vi "Motor_Initialization.vi"() -> ()   [LabVIEW 2018]
uses:
  <vilib>/Rock Robotics/WPI/ThirdParty/Phoenix-LabVIEW/Motor Controller/Controls/CTRE_Phoenix_MotorControl_ControlMode.ctl
  <vilib>/Rock Robotics/WPI/ThirdParty/Phoenix-LabVIEW/Motor Controller/Controls/CTRE_Phoenix_MotorControl_FeedbackDevice.ctl
  Global_Variables/Drive_Globals.vi
  Global_Variables/Elevator_Globals.vi
  <vilib>/Rock Robotics/WPI/ThirdParty/Phoenix-LabVIEW/Pigeon IMU/CTRE_PigeonIMU_Open_TalonSRX.vi
  Global_Variables/Climb_Globals.vi
  Global_Variables/Intake_Joint_Globals.vi
  Global_Variables/Intake_Ball_Globals.vi
panel:
  in  "D_Right":dbl
  in  "P_Right":dbl=3.0
  in  "D":dbl
  in  "P_Drive":dbl=3.0
  in  "secondsFromNeutralToFull":dbl
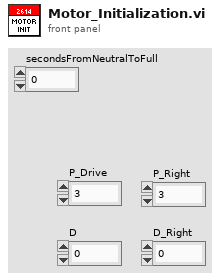
[diagram p1: front panel]
types:
  T1 = typedef "CTRE_Phoenix_MotorControl_FeedbackDevice.ctl" = i8
  T2 = typedef "CTRE_Phoenix_MotorControl_ControlMode.ctl" = u16
  T3 = enum16{"FollowerType_PercentOutput", "FollowerType_AuxOutput1"}
  T4 = typedef "WPI_MotorControlDeviceRef.ctl" = cluster{"DeviceStatus":errorcluster, "Type":T5, "PWM":cluster{"PWM Channel":T6, "DeadBand":T7}, "CAN":cluster{"Device Number":u8, "SetOutput VI Ref":variant, "GetOutput VI Ref":variant, "Enable VI Ref":variant, "Disable VI Ref":variant, "Data":variant}, "Invert":bool, "DIO PWM":cluster{"PWM \"Enable\" Channel":T6, "DIOChannel":T8, "PWM Rate":dbl}}
  T5 = typedef "WPI_MotorControlType.ctl" = enum16{"PWM", "CAN", "DIO PWM"}
  T6 = typedef "FPGA_DIOPWMChannel.ctl" = enum8{"PWM 0", "PWM 1", "PWM 2", "PWM 3", "PWM 4", "PWM 5", "PWM 6", "PWM 7", "PWM 8", "PWM 9", "PWM MXP 0", "PWM MXP 1", "PWM MXP 2", "PWM MXP 3", "PWM MXP 4", "PWM MXP 5", "PWM MXP 6", "PWM MXP 7", "PWM MXP 8", "PWM MXP 9", "Invalid"}
  T7 = typedef "WPI_PWMDeadband.ctl" = cluster{"Name":string, "maxPositivePwm":i32, "minPositivePwm":i32, "centerPwm":i32, "maxNegativePwm":i32, "minNegativePwm":i32, "angularRange":u16}
  T8 = typedef "FPGA_DIOChannel.ctl" = enum8{"DIO 0", "DIO 1", "DIO 2", "DIO 3", "DIO 4", "DIO 5", "DIO 6", "DIO 7", "DIO 8", "DIO 9", "DIO MXP 0", "DIO MXP 1", "DIO MXP 2", "DIO MXP 3", "DIO MXP 4", "DIO MXP 5", "DIO MXP 6", "DIO MXP 7", "DIO MXP 8", "DIO MXP 9", "DIO MXP 10", "DIO MXP 11", "DIO MXP 12", "DIO MXP 13", "DIO MXP 14", "DIO MXP 15", "SPI Port CS1", "SPI Port CS2", "SPI Port CS3", "SPI Port MISO", "SPI Port MOSI", "Invalid"}
  T9 = typedef "CTRE_PigeonIMU_DeviceRef.ctl" = cluster{"DeviceStatus":errorcluster, "Device Number":u8, "Type":T10, "Device ID":u32, "Handle":u64, "UsageFrame":u32, "Library Path":path}
  T10 = typedef "CTRE_PigeonIMU_ConnectionType.ctl" = u32
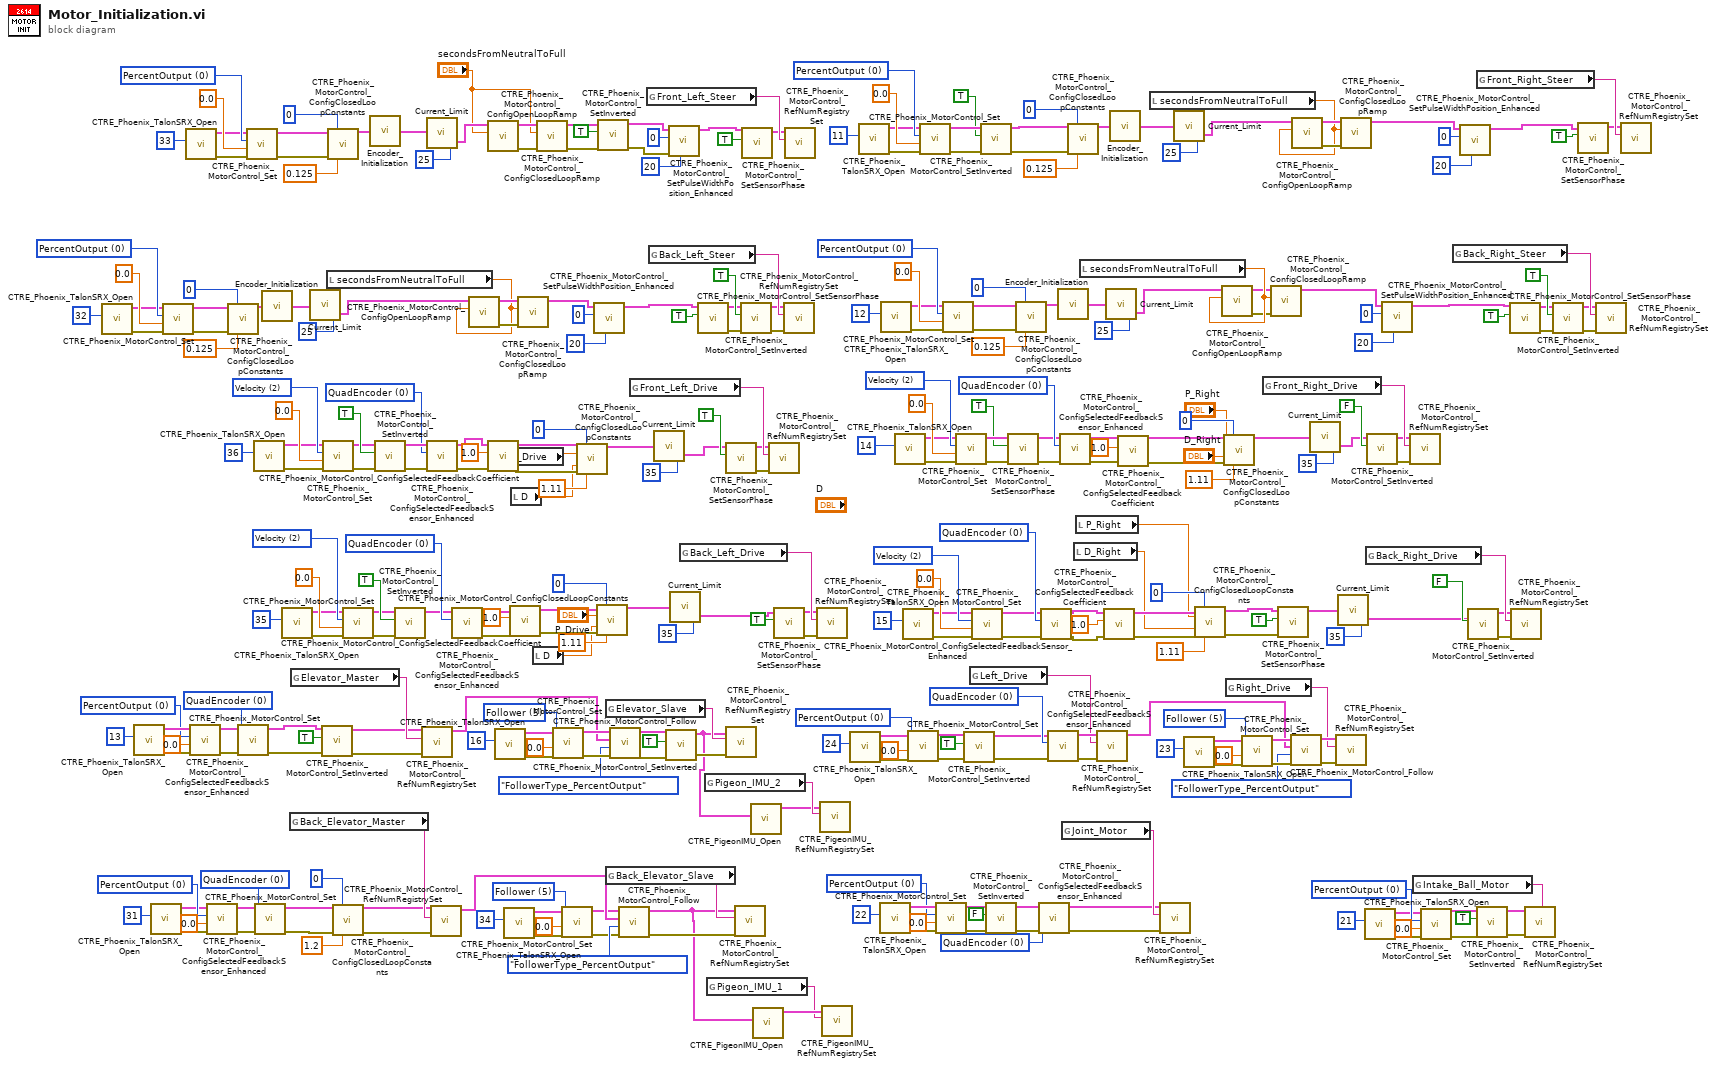
[diagram p0: block diagram]
diagram:
  w60 = T1 0 items=["QuadEncoder"=0, "Analog"=2, "Tachometer"=4, "Pulse Width Encoded Position"=8, "Sensor Sum (S0 + S1)"=9, "Sensor Difference (D0 - D1)"=10, "Remote Source 0"=11, "Remote Source 1"=12, "Software Emulated"=15] ("Feedback Device")
  w109 = T2 0 items=["PercentOutput"=0, "Position"=1, "Velocity"=2, "Current"=3, "Follower"=5, "MotionProfile"=6, "MotionMagic"=7, "MotionProfileArc"=10, "Disabled"=15] ("Control Mode")
  w114 = T2 0 items=["PercentOutput"=0, "Position"=1, "Velocity"=2, "Current"=3, "Follower"=5, "MotionProfile"=6, "MotionMagic"=7, "MotionProfileArc"=10, "Disabled"=15] ("Control Mode")
  w130 = T1 0 items=["QuadEncoder"=0, "Analog"=2, "Tachometer"=4, "Pulse Width Encoded Position"=8, "Sensor Sum (S0 + S1)"=9, "Sensor Difference (D0 - D1)"=10, "Remote Source 0"=11, "Remote Source 1"=12, "Software Emulated"=15] ("Feedback Device")
  w126 = T2 0 items=["PercentOutput"=0, "Position"=1, "Velocity"=2, "Current"=3, "Follower"=5, "MotionProfile"=6, "MotionMagic"=7, "MotionProfileArc"=10, "Disabled"=15] ("Control Mode")
  w125 = T2 5 items=["PercentOutput"=0, "Position"=1, "Velocity"=2, "Current"=3, "Follower"=5, "MotionProfile"=6, "MotionMagic"=7, "MotionProfileArc"=10, "Disabled"=15] ("Control Mode")
  w151 = T1 0 items=["None"=-1, "QuadEncoder"=0, "Analog"=2, "Tachometer"=4, "Pulse Width Encoded Position"=8, "Sensor Sum (S0 + S1)"=9, "Sensor Difference (D0 - D1)"=10, "Remote Source 0"=11, "Remote Source 1"=12, "Software Emulated"=15] ("Feedback Device")
  w154 = T2 0 items=["PercentOutput"=0, "Position"=1, "Velocity"=2, "Current"=3, "Follower"=5, "MotionProfile"=6, "MotionMagic"=7, "MotionProfileArc"=10, "Disabled"=15] ("Control Mode")
  w155 = T2 5 items=["PercentOutput"=0, "Position"=1, "Velocity"=2, "Current"=3, "Follower"=5, "MotionProfile"=6, "MotionMagic"=7, "MotionProfileArc"=10, "Disabled"=15] ("Control Mode")
  w164 = T1 0 items=["QuadEncoder"=0, "Analog"=2, "Tachometer"=4, "Pulse Width Encoded Position"=8, "Sensor Sum (S0 + S1)"=9, "Sensor Difference (D0 - D1)"=10, "Remote Source 0"=11, "Remote Source 1"=12, "Software Emulated"=15] ("Feedback Device")
  w169 = T2 0 items=["PercentOutput"=0, "Position"=1, "Velocity"=2, "Current"=3, "Follower"=5, "MotionProfile"=6, "MotionMagic"=7, "MotionProfileArc"=10, "Disabled"=15] ("Control Mode")
  w170 = T2 5 items=["PercentOutput"=0, "Position"=1, "Velocity"=2, "Current"=3, "Follower"=5, "MotionProfile"=6, "MotionMagic"=7, "MotionProfileArc"=10, "Disabled"=15] ("Control Mode")
  w214 = T1 0 items=["None"=-1, "QuadEncoder"=0, "Analog"=2, "Tachometer"=4, "Pulse Width Encoded Position"=8, "Sensor Sum (S0 + S1)"=9, "Sensor Difference (D0 - D1)"=10, "Remote Source 0"=11, "Remote Source 1"=12, "Software Emulated"=15] ("Feedback Device")
  w222 = T1 0 items=["None"=-1, "QuadEncoder"=0, "Analog"=2, "Tachometer"=4, "Pulse Width Encoded Position"=8, "Sensor Sum (S0 + S1)"=9, "Sensor Difference (D0 - D1)"=10, "Remote Source 0"=11, "Remote Source 1"=12, "Software Emulated"=15] ("Feedback Device")
  w223 = T1 0 items=["None"=-1, "QuadEncoder"=0, "Analog"=2, "Tachometer"=4, "Pulse Width Encoded Position"=8, "Sensor Sum (S0 + S1)"=9, "Sensor Difference (D0 - D1)"=10, "Remote Source 0"=11, "Remote Source 1"=12, "Software Emulated"=15] ("Feedback Device")
  w225 = T1 0 items=["None"=-1, "QuadEncoder"=0, "Analog"=2, "Tachometer"=4, "Pulse Width Encoded Position"=8, "Sensor Sum (S0 + S1)"=9, "Sensor Difference (D0 - D1)"=10, "Remote Source 0"=11, "Remote Source 1"=12, "Software Emulated"=15] ("Feedback Device")
  w246 = T2 2 items=["PercentOutput"=0, "Position"=1, "Velocity"=2, "Current"=3, "Follower"=5, "MotionProfile"=6, "MotionMagic"=7, "MotionMagicArc"=8, "MotionProfileArc"=10, "Disabled"=15] ("Control Mode")
  w251 = T2 2 items=["PercentOutput"=0, "Position"=1, "Velocity"=2, "Current"=3, "Follower"=5, "MotionProfile"=6, "MotionMagic"=7, "MotionMagicArc"=8, "MotionProfileArc"=10, "Disabled"=15] ("Control Mode")
  w256 = T2 2 items=["PercentOutput"=0, "Position"=1, "Velocity"=2, "Current"=3, "Follower"=5, "MotionProfile"=6, "MotionMagic"=7, "MotionMagicArc"=8, "MotionProfileArc"=10, "Disabled"=15] ("Control Mode")
  w261 = T2 2 items=["PercentOutput"=0, "Position"=1, "Velocity"=2, "Current"=3, "Follower"=5, "MotionProfile"=6, "MotionMagic"=7, "MotionMagicArc"=8, "MotionProfileArc"=10, "Disabled"=15] ("Control Mode")
  w293 = T2 0 items=["PercentOutput"=0, "Position"=1, "Velocity"=2, "Current"=3, "Follower"=5, "MotionProfile"=6, "MotionMagic"=7, "MotionMagicArc"=8, "MotionProfileArc"=10, "Disabled"=15] ("Control Mode")
  w302 = T2 0 items=["PercentOutput"=0, "Position"=1, "Velocity"=2, "Current"=3, "Follower"=5, "MotionProfile"=6, "MotionMagic"=7, "MotionMagicArc"=8, "MotionProfileArc"=10, "Disabled"=15] ("Control Mode")
  w311 = T2 0 items=["PercentOutput"=0, "Position"=1, "Velocity"=2, "Current"=3, "Follower"=5, "MotionProfile"=6, "MotionMagic"=7, "MotionMagicArc"=8, "MotionProfileArc"=10, "Disabled"=15] ("Control Mode")
  w320 = T2 0 items=["PercentOutput"=0, "Position"=1, "Velocity"=2, "Current"=3, "Follower"=5, "MotionProfile"=6, "MotionMagic"=7, "MotionMagicArc"=8, "MotionProfileArc"=10, "Disabled"=15] ("Control Mode")
  n1 = call <vilib>:"CTRE_Phoenix_TalonSRX_Open.vi"("Device Number"=u8 32) -> ("error out"=w313:errorcluster, "CAN Talon SRX Ref"=w310:T4)  [unwired: 9 in]
  n2 = call <vilib>:"CTRE_Phoenix_TalonSRX_Open.vi"("Device Number"=u8 13) -> ("error out"=w176:errorcluster, "CAN Talon SRX Ref"=w175:T4)  [unwired: 9 in]
  n3 = call <vilib>:"CTRE_Phoenix_TalonSRX_Open.vi"("Device Number"=u8 31) -> ("error out"=w119:errorcluster, "CAN Talon SRX Ref"=w120:T4)  [unwired: 9 in]
  n4 = call <vilib>:"CTRE_Phoenix_MotorControl_Set.vi"("error in (no error)"=w313, "Output"=0.0, "Control Mode"=w311, "PhoenixMotorControlDevRef"=w310) -> ("error out"=w315:errorcluster, "PhoenixMotorControlDevRef"=w314:T4)  [unwired: 6 in]
  n5 = call <vilib>:"CTRE_Phoenix_TalonSRX_Open.vi"("Device Number"=u8 33) -> ("error out"=w322:errorcluster, "CAN Talon SRX Ref"=w319:T4)  [unwired: 9 in]
  n6 = call <vilib>:"CTRE_Phoenix_MotorControl_Set.vi"("error in (no error)"=w176, "Output"=0.0, "Control Mode"=w169, "PhoenixMotorControlDevRef"=w175) -> ("error out"=w166:errorcluster, "PhoenixMotorControlDevRef"=w165:T4)  [unwired: 6 in]
  n7 = call <vilib>:"CTRE_Phoenix_MotorControl_Set.vi"("error in (no error)"=w119, "Output"=0.0, "Control Mode"=w126, "PhoenixMotorControlDevRef"=w120) -> ("error out"=w128:errorcluster, "PhoenixMotorControlDevRef"=w129:T4)  [unwired: 6 in]
  n8 = call <vilib>:"CTRE_Phoenix_MotorControl_ConfigClosedLoopConstants.vi"("PhoenixMotorControlDevRef"=w314, "slotIdx"=0, "error in (no error)"=w315, "F"=0.125) -> ("PhoenixMotorControlDevRef"=w279:T4)  [unwired: 10 in, 1 out]
  n9 = call <vilib>:"CTRE_Phoenix_MotorControl_ConfigSelectedFeedbackSensor_Enhanced.vi"("error in (no error)"=w166, "Feedback Device"=w164, "PhoenixMotorControlDevRef"=w165) -> ("error out"=w94:errorcluster, "PhoenixMotorControlDevRef"=w95:T4)  [unwired: 7 in]
  n10 = call <vilib>:"CTRE_Phoenix_MotorControl_Set.vi"("error in (no error)"=w322, "Output"=0.0, "Control Mode"=w320, "PhoenixMotorControlDevRef"=w319) -> ("error out"=w324:errorcluster, "PhoenixMotorControlDevRef"=w323:T4)  [unwired: 6 in]
  n11 = call <vilib>:"CTRE_Phoenix_TalonSRX_Open.vi"("Device Number"=u8 36) -> ("error out"=w206:errorcluster, "CAN Talon SRX Ref"=w207:T4)  [unwired: 9 in]
  n12 = call <vilib>:"CTRE_Phoenix_MotorControl_ConfigSelectedFeedbackSensor_Enhanced.vi"("error in (no error)"=w128, "Feedback Device"=w130, "PhoenixMotorControlDevRef"=w129) -> ("error out"=w86:errorcluster, "PhoenixMotorControlDevRef"=w87:T4)  [unwired: 7 in]
  n13 = call "Encoder_Initialization.vi"("Ref In"=w279) -> ("Ref Out"=w78:T4)  [unwired: 1 in]
  n14 = call <vilib>:"CTRE_Phoenix_TalonSRX_Open.vi"("Device Number"=u8 35) -> ("error out"=w248:errorcluster, "CAN Talon SRX Ref"=w245:T4)  [unwired: 9 in]
  n15 = global read "Climb_Globals.vi" "Back_Elevator_Master"() -> (w118:string)
  n16 = global read "Elevator_Globals.vi" "Elevator_Master"() -> (w167:string)
  n17 = call "Current_Limit.vi"("Ref In"=w78, "Current_Limit"=25) -> ("Ref Out"=w38:T4)
  n18 = call <vilib>:"CTRE_Phoenix_MotorControl_SetInverted.vi"("error in (no error)"=w94, "Invert?"=TRUE, "PhoenixMotorControlDevRef"=w95) -> ("error out"=w92:errorcluster, "PhoenixMotorControlDevRef"=w93:T4)  [unwired: 7 in]
  n19 = call <vilib>:"CTRE_Phoenix_MotorControl_Set.vi"("error in (no error)"=w206, "Output"=0.0, "Control Mode"=w251, "PhoenixMotorControlDevRef"=w207) -> ("error out"=w241:errorcluster, "PhoenixMotorControlDevRef"=w242:T4)  [unwired: 6 in]
  n20 = local read "secondsFromNeutralToFull"() -> (w39:dbl)
  n21 = call <vilib>:"CTRE_Phoenix_MotorControl_ConfigClosedLoopConstants.vi"("PhoenixMotorControlDevRef"=w323, "slotIdx"=0, "error in (no error)"=w324, "F"=0.125) -> ("PhoenixMotorControlDevRef"=w282:T4)  [unwired: 10 in, 1 out]
  n22 = call <vilib>:"CTRE_Phoenix_MotorControl_ConfigClosedLoopConstants.vi"("PhoenixMotorControlDevRef"=w87, "slotIdx"=0, "error in (no error)"=w86, "F"=1.2) -> ("PhoenixMotorControlDevRef"=w85:T4, "error out"=w84:errorcluster)  [unwired: 10 in]
  n23 = call <vilib>:"CTRE_Phoenix_MotorControl_Set.vi"("error in (no error)"=w248, "Output"=0.0, "Control Mode"=w246, "PhoenixMotorControlDevRef"=w245) -> ("error out"=w238:errorcluster, "PhoenixMotorControlDevRef"=w239:T4)  [unwired: 6 in]
  n24 = call "Encoder_Initialization.vi"("Ref In"=w282) -> ("Ref Out"=w77:T4)  [unwired: 1 in]
  n25 = call <vilib>:"CTRE_Phoenix_MotorControl_SetInverted.vi"("error in (no error)"=w241, "Invert?"=TRUE, "PhoenixMotorControlDevRef"=w242) -> ("error out"=w218:errorcluster, "PhoenixMotorControlDevRef"=w217:T4)  [unwired: 7 in]
  n26 = call <vilib>:"CTRE_Phoenix_MotorControl_SetInverted.vi"("error in (no error)"=w238, "Invert?"=TRUE, "PhoenixMotorControlDevRef"=w239) -> ("PhoenixMotorControlDevRef"=w224:T4)  [unwired: 7 in, 1 out]
  n27 = call <vilib>:"CTRE_Phoenix_MotorControl_RefNumRegistrySet.vi"("error in (no error)"=w92, "refnum name"=w167, "PhoenixMotorControlDevRef"=w93) -> ("PhoenixMotorControlDevRef"=w139:T4)  [unwired: 7 in, 1 out]
  n28 = call "Current_Limit.vi"("Ref In"=w77, "Current_Limit"=25) -> ("Ref Out"=w43:T4)
  n29 = call <vilib>:"CTRE_Phoenix_MotorControl_ConfigSelectedFeedbackSensor_Enhanced.vi"("error in (no error)"=w218, "Feedback Device"=w214, "PhoenixMotorControlDevRef"=w217) -> ("error out"=w181:errorcluster, "PhoenixMotorControlDevRef"=w182:T4)  [unwired: 7 in]
  n30 = call <vilib>:"CTRE_Phoenix_MotorControl_RefNumRegistrySet.vi"("error in (no error)"=w84, "refnum name"=w118, "PhoenixMotorControlDevRef"=w85) -> ("PhoenixMotorControlDevRef"=w136:T4)  [unwired: 7 in, 1 out]
  n31 = call <vilib>:"CTRE_Phoenix_MotorControl_ConfigSelectedFeedbackSensor_Enhanced.vi"("Feedback Device"=w225, "PhoenixMotorControlDevRef"=w224) -> ("error out"=w208:errorcluster, "PhoenixMotorControlDevRef"=w209:T4)  [unwired: 8 in]
  n32 = call <vilib>:"CTRE_Phoenix_MotorControl_ConfigOpenLoopRamp.vi"("secondsFromNeutralToFull"=w39, "PhoenixMotorControlDevRef"=w38) -> ("error out"=w41:errorcluster, "PhoenixMotorControlDevRef"=w40:T4)  [unwired: 8 in]
  n33 = call <vilib>:"CTRE_Phoenix_MotorControl_ConfigOpenLoopRamp.vi"("secondsFromNeutralToFull"="secondsFromNeutralToFull", "PhoenixMotorControlDevRef"=w43) -> ("error out"=w44:errorcluster, "PhoenixMotorControlDevRef"=w45:T4)  [unwired: 8 in]
  n34 = call <vilib>:"CTRE_Phoenix_MotorControl_ConfigSelectedFeedbackCoefficient.vi"("error in (no error)"=w181, "coefficient"=1.0, "PhoenixMotorControlDevRef"=w182) -> ("error out"=w177:errorcluster, "PhoenixMotorControlDevRef"=w178:T4)  [unwired: 7 in]
  n35 = call <vilib>:"CTRE_Phoenix_TalonSRX_Open.vi"("Device Number"=u8 16) -> ("error out"=w174:errorcluster, "CAN Talon SRX Ref"=w173:T4)  [unwired: 9 in]
  n36 = local read "P_Drive"() -> (w12:dbl)
  n37 = call <vilib>:"CTRE_Phoenix_TalonSRX_Open.vi"("Device Number"=u8 34) -> ("error out"=w121:errorcluster, "CAN Talon SRX Ref"=w122:T4)  [unwired: 9 in]
  n38 = call <vilib>:"CTRE_Phoenix_MotorControl_ConfigSelectedFeedbackCoefficient.vi"("error in (no error)"=w208, "coefficient"=1.0, "PhoenixMotorControlDevRef"=w209) -> ("error out"=w184:errorcluster, "PhoenixMotorControlDevRef"=w185:T4)  [unwired: 7 in]
  n39 = local read "D"() -> (w5:dbl)
  n40 = call <vilib>:"CTRE_Phoenix_MotorControl_ConfigClosedLoopRamp.vi"("error in (no error)"=w41, "secondsFromNeutralToFull"=w39, "PhoenixMotorControlDevRef"=w40) -> ("PhoenixMotorControlDevRef"=w37:T4)  [unwired: 7 in, 1 out]
  n41 = local read "D"() -> (w6:dbl)
  n42 = call <vilib>:"CTRE_Phoenix_MotorControl_ConfigClosedLoopRamp.vi"("error in (no error)"=w44, "secondsFromNeutralToFull"="secondsFromNeutralToFull", "PhoenixMotorControlDevRef"=w45) -> ("error out"=w25:errorcluster, "PhoenixMotorControlDevRef"=w26:T4)  [unwired: 7 in]
  n43 = call <vilib>:"CTRE_Phoenix_MotorControl_Set.vi"("error in (no error)"=w174, "Output"=0.0, "Control Mode"=w170, "PhoenixMotorControlDevRef"=w173) -> ("error out"=w172:errorcluster, "PhoenixMotorControlDevRef"=w171:T4)  [unwired: 6 in]
  n44 = call <vilib>:"CTRE_Phoenix_MotorControl_Set.vi"("error in (no error)"=w121, "Output"=0.0, "Control Mode"=w125, "PhoenixMotorControlDevRef"=w122) -> ("error out"=w123:errorcluster, "PhoenixMotorControlDevRef"=w124:T4)  [unwired: 6 in]
  n45 = call <vilib>:"CTRE_Phoenix_MotorControl_ConfigClosedLoopConstants.vi"("PhoenixMotorControlDevRef"=w178, "slotIdx"=0, "P"=w12, "D"=w5, "error in (no error)"=w177, "F"=1.11) -> ("PhoenixMotorControlDevRef"=w70:T4)  [unwired: 8 in, 1 out]
  n46 = call <vilib>:"CTRE_Phoenix_MotorControl_SetPulseWidthPosition_Enhanced.vi"("timeoutMs"=u32 20, "New Position"=0, "PhoenixMotorControlDevRef"=w37) -> ("PhoenixMotorControlDevRef"=w66:T4)  [unwired: 7 in, 1 out]
  n47 = call <vilib>:"CTRE_Phoenix_MotorControl_ConfigClosedLoopConstants.vi"("PhoenixMotorControlDevRef"=w185, "slotIdx"=0, "P"="P_Drive", "D"=w6, "error in (no error)"=w184, "F"=1.11) -> ("PhoenixMotorControlDevRef"=w72:T4)  [unwired: 8 in, 1 out]
  n48 = call <vilib>:"CTRE_Phoenix_MotorControl_SetInverted.vi"("error in (no error)"=w25, "Invert?"=TRUE, "PhoenixMotorControlDevRef"=w26) -> ("error out"=w23:errorcluster, "PhoenixMotorControlDevRef"=w24:T4)  [unwired: 7 in]
  n49 = global read "Elevator_Globals.vi" "Elevator_Slave"() -> (w168:string)
  n50 = global read "Climb_Globals.vi" "Back_Elevator_Slave"() -> (w117:string)
  n51 = call <vilib>:"CTRE_Phoenix_MotorControl_Follow.vi"("error in (no error)"=w172, "FollowerType"=T3."FollowerType_PercentOutput", "Master Controller to Follow"=w139, "PhoenixMotorControlDevRef"=w171) -> ("error out"=w88:errorcluster, "PhoenixMotorControlDevRef"=w90:T4)  [unwired: 6 in]
  n52 = call <vilib>:"CTRE_Phoenix_MotorControl_Follow.vi"("error in (no error)"=w123, "FollowerType"=T3."FollowerType_PercentOutput", "Master Controller to Follow"=w136, "PhoenixMotorControlDevRef"=w124) -> ("error out"=w127:errorcluster, "PhoenixMotorControlDevRef"=w46:T4)  [unwired: 6 in]
  n53 = global read "Drive_Globals.vi" "Front_Left_Drive"() -> (w253:string)
  n54 = global read "Drive_Globals.vi" "Front_Left_Steer"() -> (w286:string)
  n55 = global read "Drive_Globals.vi" "Back_Left_Steer"() -> (w317:string)
  n56 = call "Current_Limit.vi"("Ref In"=w70, "Current_Limit"=35) -> ("Ref Out"=w69:T4)
  n57 = call <vilib>:"CTRE_Phoenix_MotorControl_SetInverted.vi"("error in (no error)"=w88, "Invert?"=TRUE, "PhoenixMotorControlDevRef"=w90) -> ("error out"=w89:errorcluster, "PhoenixMotorControlDevRef"=w49:T4)  [unwired: 7 in]
  n58 = call <vilib>:"CTRE_Phoenix_MotorControl_SetPulseWidthPosition_Enhanced.vi"("timeoutMs"=u32 20, "error in (no error)"=w23, "New Position"=0, "PhoenixMotorControlDevRef"=w24) -> ("PhoenixMotorControlDevRef"=w65:T4)  [unwired: 6 in, 1 out]
  n59 = call "Current_Limit.vi"("Ref In"=w72, "Current_Limit"=35) -> ("Ref Out"=w71:T4)
  n60 = global read "Drive_Globals.vi" "Back_Left_Drive"() -> (w249:string)
  n61 = call <vilib>:"CTRE_Phoenix_MotorControl_SetSensorPhase.vi"("PhaseSensor"=TRUE, "PhoenixMotorControlDevRef"=w66) -> ("error out"=w266:errorcluster, "PhoenixMotorControlDevRef"=w267:T4)  [unwired: 8 in]
  n62 = global read "Drive_Globals.vi" "Pigeon_IMU_2"() -> (w51:string)
  n63 = global read "Drive_Globals.vi" "Pigeon_IMU_1"() -> (w47:string)
  n64 = call <vilib>:"CTRE_Phoenix_MotorControl_SetSensorPhase.vi"("PhaseSensor"=TRUE, "PhoenixMotorControlDevRef"=w69) -> ("error out"=w215:errorcluster, "PhoenixMotorControlDevRef"=w216:T4)  [unwired: 8 in]
  n65 = call <vilib>:"CTRE_Phoenix_MotorControl_RefNumRegistrySet.vi"("error in (no error)"=w89, "refnum name"=w168, "PhoenixMotorControlDevRef"=w49) -> ()  [unwired: 7 in, 2 out]
  n66 = call <vilib>:"CTRE_Phoenix_MotorControl_RefNumRegistrySet.vi"("error in (no error)"=w127, "refnum name"=w117, "PhoenixMotorControlDevRef"=w46) -> ()  [unwired: 7 in, 2 out]
  n67 = call <vilib>:"CTRE_Phoenix_MotorControl_SetInverted.vi"("error in (no error)"=w266, "Invert?"=TRUE, "PhoenixMotorControlDevRef"=w267) -> ("error out"=w265:errorcluster, "PhoenixMotorControlDevRef"=w264:T4)  [unwired: 7 in]
  n68 = call <vilib>:"CTRE_Phoenix_MotorControl_SetSensorPhase.vi"("PhaseSensor"=TRUE, "PhoenixMotorControlDevRef"=w65) -> ("PhoenixMotorControlDevRef"=w277:T4)  [unwired: 8 in, 1 out]
  n69 = call-poly <vilib>:"CTRE_PigeonIMU_Open.vi"("CAN Talon SRX Ref"=w49) -> ("PigeonIMUDevRef"=w50:T9)  [unwired: 9 in, 1 out]
  n70 = call-poly <vilib>:"CTRE_PigeonIMU_Open.vi"("CAN Talon SRX Ref"=w46) -> ("PigeonIMUDevRef"=w48:T9)  [unwired: 9 in, 1 out]
  n71 = call <vilib>:"CTRE_Phoenix_MotorControl_RefNumRegistrySet.vi"("error in (no error)"=w215, "refnum name"=w253, "PhoenixMotorControlDevRef"=w216) -> ()  [unwired: 7 in, 2 out]
  n72 = call <vilib>:"CTRE_Phoenix_MotorControl_SetSensorPhase.vi"("PhaseSensor"=TRUE, "PhoenixMotorControlDevRef"=w71) -> ("error out"=w230:errorcluster, "PhoenixMotorControlDevRef"=w231:T4)  [unwired: 8 in]
  n73 = call <vilib>:"CTRE_Phoenix_MotorControl_RefNumRegistrySet.vi"("error in (no error)"=w265, "refnum name"=w317, "PhoenixMotorControlDevRef"=w264) -> ()  [unwired: 7 in, 2 out]
  n74 = call <vilib>:"CTRE_Phoenix_MotorControl_RefNumRegistrySet.vi"("refnum name"=w286, "PhoenixMotorControlDevRef"=w277) -> ()  [unwired: 8 in, 2 out]
  n75 = call <vilib>:"CTRE_Phoenix_MotorControl_RefNumRegistrySet.vi"("error in (no error)"=w230, "refnum name"=w249, "PhoenixMotorControlDevRef"=w231) -> ()  [unwired: 7 in, 2 out]
  n76 = call <vilib>:"CTRE_PigeonIMU_RefNumRegistrySet.vi"("refnum name"=w51, "PigeonIMUDevRef"=w50) -> ()  [unwired: 8 in, 2 out]
  n77 = call <vilib>:"CTRE_PigeonIMU_RefNumRegistrySet.vi"("refnum name"=w47, "PigeonIMUDevRef"=w48) -> ()  [unwired: 8 in, 2 out]
  n78 = call <vilib>:"CTRE_Phoenix_TalonSRX_Open.vi"("Device Number"=u8 24) -> ("error out"=w159:errorcluster, "CAN Talon SRX Ref"=w160:T4)  [unwired: 9 in]
  n79 = call <vilib>:"CTRE_Phoenix_TalonSRX_Open.vi"("Device Number"=u8 11) -> ("error out"=w304:errorcluster, "CAN Talon SRX Ref"=w301:T4)  [unwired: 9 in]
  n80 = call <vilib>:"CTRE_Phoenix_TalonSRX_Open.vi"("Device Number"=u8 22) -> ("error out"=w116:errorcluster, "CAN Talon SRX Ref"=w115:T4)  [unwired: 9 in]
  n81 = call <vilib>:"CTRE_Phoenix_TalonSRX_Open.vi"("Device Number"=u8 12) -> ("error out"=w295:errorcluster, "CAN Talon SRX Ref"=w292:T4)  [unwired: 9 in]
  n82 = call <vilib>:"CTRE_Phoenix_TalonSRX_Open.vi"("Device Number"=u8 14) -> ("error out"=w211:errorcluster, "CAN Talon SRX Ref"=w212:T4)  [unwired: 9 in]
  n83 = call <vilib>:"CTRE_Phoenix_TalonSRX_Open.vi"("Device Number"=u8 15) -> ("error out"=w258:errorcluster, "CAN Talon SRX Ref"=w255:T4)  [unwired: 9 in]
  n84 = call <vilib>:"CTRE_Phoenix_MotorControl_Set.vi"("error in (no error)"=w159, "Output"=0.0, "Control Mode"=w154, "PhoenixMotorControlDevRef"=w160) -> ("error out"=w101:errorcluster, "PhoenixMotorControlDevRef"=w100:T4)  [unwired: 6 in]
  n85 = call <vilib>:"CTRE_Phoenix_MotorControl_Set.vi"("error in (no error)"=w304, "Output"=0.0, "Control Mode"=w302, "PhoenixMotorControlDevRef"=w301) -> ("error out"=w306:errorcluster, "PhoenixMotorControlDevRef"=w305:T4)  [unwired: 6 in]
  n86 = call <vilib>:"CTRE_Phoenix_MotorControl_Set.vi"("error in (no error)"=w116, "Output"=0.0, "Control Mode"=w114, "PhoenixMotorControlDevRef"=w115) -> ("error out"=w104:errorcluster, "PhoenixMotorControlDevRef"=w103:T4)  [unwired: 6 in]
  n87 = call <vilib>:"CTRE_Phoenix_MotorControl_Set.vi"("error in (no error)"=w295, "Output"=0.0, "Control Mode"=w293, "PhoenixMotorControlDevRef"=w292) -> ("error out"=w297:errorcluster, "PhoenixMotorControlDevRef"=w296:T4)  [unwired: 6 in]
  n88 = call <vilib>:"CTRE_Phoenix_MotorControl_Set.vi"("error in (no error)"=w211, "Output"=0.0, "Control Mode"=w261, "PhoenixMotorControlDevRef"=w212) -> ("error out"=w228:errorcluster, "PhoenixMotorControlDevRef"=w227:T4)  [unwired: 6 in]
  n89 = call <vilib>:"CTRE_Phoenix_MotorControl_SetInverted.vi"("error in (no error)"=w101, "Invert?"=TRUE, "PhoenixMotorControlDevRef"=w100) -> ("error out"=w98:errorcluster, "PhoenixMotorControlDevRef"=w99:T4)  [unwired: 7 in]
  n90 = global read "Climb_Globals.vi" "Left_Drive"() -> (w142:string)
  n91 = call <vilib>:"CTRE_Phoenix_MotorControl_Set.vi"("error in (no error)"=w258, "Output"=0.0, "Control Mode"=w256, "PhoenixMotorControlDevRef"=w255) -> ("error out"=w196:errorcluster, "PhoenixMotorControlDevRef"=w197:T4)  [unwired: 6 in]
  n92 = call <vilib>:"CTRE_Phoenix_MotorControl_SetInverted.vi"("error in (no error)"=w306, "Invert?"=TRUE, "PhoenixMotorControlDevRef"=w305) -> ("error out"=w284:errorcluster, "PhoenixMotorControlDevRef"=w283:T4)  [unwired: 7 in]
  n93 = call <vilib>:"CTRE_Phoenix_MotorControl_SetInverted.vi"("error in (no error)"=w104, "Invert?"=FALSE, "PhoenixMotorControlDevRef"=w103) -> ("error out"=w64:errorcluster, "PhoenixMotorControlDevRef"=w63:T4)  [unwired: 7 in]
  n94 = call <vilib>:"CTRE_Phoenix_MotorControl_SetSensorPhase.vi"("error in (no error)"=w228, "PhaseSensor"=TRUE, "PhoenixMotorControlDevRef"=w227) -> ("error out"=w220:errorcluster, "PhoenixMotorControlDevRef"=w221:T4)  [unwired: 7 in]
  n95 = call <vilib>:"CTRE_Phoenix_MotorControl_ConfigClosedLoopConstants.vi"("PhoenixMotorControlDevRef"=w296, "slotIdx"=0, "error in (no error)"=w297, "F"=0.125) -> ("PhoenixMotorControlDevRef"=w281:T4)  [unwired: 10 in, 1 out]
  n96 = call <vilib>:"CTRE_Phoenix_MotorControl_ConfigSelectedFeedbackSensor_Enhanced.vi"("error in (no error)"=w64, "Feedback Device"=w60, "PhoenixMotorControlDevRef"=w63) -> ("error out"=w61:errorcluster, "PhoenixMotorControlDevRef"=w62:T4)  [unwired: 7 in]
  n97 = call <vilib>:"CTRE_Phoenix_MotorControl_ConfigSelectedFeedbackSensor_Enhanced.vi"("error in (no error)"=w196, "Feedback Device"=w223, "PhoenixMotorControlDevRef"=w197) -> ("error out"=w194:errorcluster, "PhoenixMotorControlDevRef"=w195:T4)  [unwired: 7 in]
  n98 = call <vilib>:"CTRE_Phoenix_MotorControl_ConfigSelectedFeedbackSensor_Enhanced.vi"("error in (no error)"=w98, "Feedback Device"=w151, "PhoenixMotorControlDevRef"=w99) -> ("error out"=w146:errorcluster, "PhoenixMotorControlDevRef"=w145:T4)  [unwired: 7 in]
  n99 = call "Encoder_Initialization.vi"("Ref In"=w281) -> ("Ref Out"=w80:T4)  [unwired: 1 in]
  n100 = call <vilib>:"CTRE_Phoenix_MotorControl_ConfigSelectedFeedbackSensor_Enhanced.vi"("error in (no error)"=w220, "Feedback Device"=w222, "PhoenixMotorControlDevRef"=w221) -> ("error out"=w203:errorcluster, "PhoenixMotorControlDevRef"=w204:T4)  [unwired: 7 in]
  n101 = global read "Intake_Joint_Globals.vi" "Joint_Motor"() -> (w106:string)
  n102 = call <vilib>:"CTRE_Phoenix_MotorControl_ConfigClosedLoopConstants.vi"("PhoenixMotorControlDevRef"=w283, "slotIdx"=0, "error in (no error)"=w284, "F"=0.125) -> ("PhoenixMotorControlDevRef"=w280:T4)  [unwired: 10 in, 1 out]
  n103 = local read "D_Right"() -> (w2:dbl)
  n104 = local read "P_Right"() -> (w1:dbl)
  n105 = local read "secondsFromNeutralToFull"() -> (w36:dbl)
  n106 = call <vilib>:"CTRE_Phoenix_MotorControl_RefNumRegistrySet.vi"("error in (no error)"=w146, "refnum name"=w142, "PhoenixMotorControlDevRef"=w145) -> ("PhoenixMotorControlDevRef"=w140:T4)  [unwired: 7 in, 1 out]
  n107 = call <vilib>:"CTRE_Phoenix_MotorControl_ConfigSelectedFeedbackCoefficient.vi"("error in (no error)"=w194, "coefficient"=1.0, "PhoenixMotorControlDevRef"=w195) -> ("error out"=w190:errorcluster, "PhoenixMotorControlDevRef"=w191:T4)  [unwired: 7 in]
  n108 = call "Current_Limit.vi"("Ref In"=w80, "Current_Limit"=25) -> ("Ref Out"=w33:T4)
  n109 = call "Encoder_Initialization.vi"("Ref In"=w280) -> ("Ref Out"=w79:T4)  [unwired: 1 in]
  n110 = call <vilib>:"CTRE_Phoenix_MotorControl_ConfigSelectedFeedbackCoefficient.vi"("error in (no error)"=w203, "coefficient"=1.0, "PhoenixMotorControlDevRef"=w204) -> ("error out"=w199:errorcluster, "PhoenixMotorControlDevRef"=w200:T4)  [unwired: 7 in]
  n111 = local read "secondsFromNeutralToFull"() -> (w29:dbl)
  n112 = call <vilib>:"CTRE_Phoenix_MotorControl_RefNumRegistrySet.vi"("error in (no error)"=w61, "refnum name"=w106, "PhoenixMotorControlDevRef"=w62) -> ()  [unwired: 7 in, 2 out]
  n113 = call "Current_Limit.vi"("Ref In"=w79, "Current_Limit"=25) -> ("Ref Out"=w28:T4)
  n114 = call <vilib>:"CTRE_Phoenix_TalonSRX_Open.vi"("Device Number"=u8 23) -> ("error out"=w158:errorcluster, "CAN Talon SRX Ref"=w157:T4)  [unwired: 9 in]
  n115 = call <vilib>:"CTRE_Phoenix_MotorControl_ConfigClosedLoopConstants.vi"("PhoenixMotorControlDevRef"=w191, "slotIdx"=0, "P"=w1, "D"=w2, "error in (no error)"=w190, "F"=1.11) -> ("PhoenixMotorControlDevRef"=w188:T4, "error out"=w189:errorcluster)  [unwired: 8 in]
  n116 = call <vilib>:"CTRE_Phoenix_MotorControl_ConfigOpenLoopRamp.vi"("secondsFromNeutralToFull"=w36, "PhoenixMotorControlDevRef"=w33) -> ("error out"=w34:errorcluster, "PhoenixMotorControlDevRef"=w35:T4)  [unwired: 8 in]
  n117 = call <vilib>:"CTRE_Phoenix_MotorControl_ConfigClosedLoopConstants.vi"("PhoenixMotorControlDevRef"=w200, "slotIdx"=0, "P"="P_Right", "D"="D_Right", "error in (no error)"=w199, "F"=1.11) -> ("PhoenixMotorControlDevRef"=w74:T4)  [unwired: 8 in, 1 out]
  n118 = global read "Climb_Globals.vi" "Right_Drive"() -> (w141:string)
  n119 = call <vilib>:"CTRE_Phoenix_MotorControl_Set.vi"("error in (no error)"=w158, "Output"=0.0, "Control Mode"=w155, "PhoenixMotorControlDevRef"=w157) -> ("error out"=w150:errorcluster, "PhoenixMotorControlDevRef"=w149:T4)  [unwired: 6 in]
  n120 = global read "Drive_Globals.vi" "Front_Right_Drive"() -> (w263:string)
  n121 = call <vilib>:"CTRE_Phoenix_MotorControl_ConfigClosedLoopRamp.vi"("error in (no error)"=w34, "secondsFromNeutralToFull"=w36, "PhoenixMotorControlDevRef"=w35) -> ("PhoenixMotorControlDevRef"=w32:T4)  [unwired: 7 in, 1 out]
  n122 = call <vilib>:"CTRE_Phoenix_MotorControl_SetSensorPhase.vi"("error in (no error)"=w189, "PhaseSensor"=TRUE, "PhoenixMotorControlDevRef"=w188) -> ("PhoenixMotorControlDevRef"=w76:T4)  [unwired: 7 in, 1 out]
  n123 = call <vilib>:"CTRE_Phoenix_MotorControl_Follow.vi"("error in (no error)"=w150, "FollowerType"=T3."FollowerType_PercentOutput", "Master Controller to Follow"=w140, "PhoenixMotorControlDevRef"=w149) -> ("error out"=w144:errorcluster, "PhoenixMotorControlDevRef"=w143:T4)  [unwired: 6 in]
  n124 = call <vilib>:"CTRE_Phoenix_MotorControl_ConfigOpenLoopRamp.vi"("secondsFromNeutralToFull"=w29, "PhoenixMotorControlDevRef"=w28) -> ("error out"=w31:errorcluster, "PhoenixMotorControlDevRef"=w30:T4)  [unwired: 8 in]
  n125 = call "Current_Limit.vi"("Ref In"=w74, "Current_Limit"=35) -> ("Ref Out"=w73:T4)
  n126 = call <vilib>:"CTRE_Phoenix_MotorControl_RefNumRegistrySet.vi"("error in (no error)"=w144, "refnum name"=w141, "PhoenixMotorControlDevRef"=w143) -> ()  [unwired: 7 in, 2 out]
  n127 = call "Current_Limit.vi"("Ref In"=w76, "Current_Limit"=35) -> ("Ref Out"=w75:T4)
  n128 = call <vilib>:"CTRE_Phoenix_MotorControl_ConfigClosedLoopRamp.vi"("error in (no error)"=w31, "secondsFromNeutralToFull"=w29, "PhoenixMotorControlDevRef"=w30) -> ("PhoenixMotorControlDevRef"=w27:T4)  [unwired: 7 in, 1 out]
  n129 = call <vilib>:"CTRE_Phoenix_TalonSRX_Open.vi"("Device Number"=u8 21) -> ("error out"=w107:errorcluster, "CAN Talon SRX Ref"=w108:T4)  [unwired: 9 in]
  n130 = global read "Drive_Globals.vi" "Back_Right_Drive"() -> (w259:string)
  n131 = call <vilib>:"CTRE_Phoenix_MotorControl_SetInverted.vi"("Invert?"=FALSE, "PhoenixMotorControlDevRef"=w73) -> ("error out"=w234:errorcluster, "PhoenixMotorControlDevRef"=w233:T4)  [unwired: 8 in]
  n132 = call <vilib>:"CTRE_Phoenix_MotorControl_SetPulseWidthPosition_Enhanced.vi"("timeoutMs"=u32 20, "New Position"=0, "PhoenixMotorControlDevRef"=w32) -> ("PhoenixMotorControlDevRef"=w67:T4)  [unwired: 7 in, 1 out]
  n133 = call <vilib>:"CTRE_Phoenix_MotorControl_RefNumRegistrySet.vi"("error in (no error)"=w234, "refnum name"=w263, "PhoenixMotorControlDevRef"=w233) -> ()  [unwired: 7 in, 2 out]
  n134 = global read "Intake_Ball_Globals.vi" "Intake_Ball_Motor"() -> (w105:string)
  n135 = call <vilib>:"CTRE_Phoenix_MotorControl_Set.vi"("error in (no error)"=w107, "Output"=0.0, "Control Mode"=w109, "PhoenixMotorControlDevRef"=w108) -> ("error out"=w10:errorcluster, "PhoenixMotorControlDevRef"=w11:T4)  [unwired: 6 in]
  n136 = global read "Drive_Globals.vi" "Back_Right_Steer"() -> (w299:string)
  n137 = call <vilib>:"CTRE_Phoenix_MotorControl_SetPulseWidthPosition_Enhanced.vi"("timeoutMs"=u32 20, "New Position"=0, "PhoenixMotorControlDevRef"=w27) -> ("PhoenixMotorControlDevRef"=w68:T4)  [unwired: 7 in, 1 out]
  n138 = call <vilib>:"CTRE_Phoenix_MotorControl_SetInverted.vi"("Invert?"=FALSE, "PhoenixMotorControlDevRef"=w75) -> ("error out"=w236:errorcluster, "PhoenixMotorControlDevRef"=w235:T4)  [unwired: 8 in]
  n139 = global read "Drive_Globals.vi" "Front_Right_Steer"() -> (w308:string)
  n140 = call <vilib>:"CTRE_Phoenix_MotorControl_SetInverted.vi"("error in (no error)"=w10, "Invert?"=TRUE, "PhoenixMotorControlDevRef"=w11) -> ("error out"=w9:errorcluster, "PhoenixMotorControlDevRef"=w8:T4)  [unwired: 7 in]
  n141 = call <vilib>:"CTRE_Phoenix_MotorControl_SetSensorPhase.vi"("PhaseSensor"=TRUE, "PhoenixMotorControlDevRef"=w67) -> ("error out"=w271:errorcluster, "PhoenixMotorControlDevRef"=w272:T4)  [unwired: 8 in]
  n142 = call <vilib>:"CTRE_Phoenix_MotorControl_RefNumRegistrySet.vi"("error in (no error)"=w236, "refnum name"=w259, "PhoenixMotorControlDevRef"=w235) -> ()  [unwired: 7 in, 2 out]
  n143 = call <vilib>:"CTRE_Phoenix_MotorControl_RefNumRegistrySet.vi"("error in (no error)"=w9, "refnum name"=w105, "PhoenixMotorControlDevRef"=w8) -> ()  [unwired: 7 in, 2 out]
  n144 = call <vilib>:"CTRE_Phoenix_MotorControl_SetInverted.vi"("error in (no error)"=w271, "Invert?"=TRUE, "PhoenixMotorControlDevRef"=w272) -> ("error out"=w270:errorcluster, "PhoenixMotorControlDevRef"=w269:T4)  [unwired: 7 in]
  n145 = call <vilib>:"CTRE_Phoenix_MotorControl_SetSensorPhase.vi"("PhaseSensor"=TRUE, "PhoenixMotorControlDevRef"=w68) -> ("PhoenixMotorControlDevRef"=w275:T4)  [unwired: 8 in, 1 out]
  n146 = call <vilib>:"CTRE_Phoenix_MotorControl_RefNumRegistrySet.vi"("error in (no error)"=w270, "refnum name"=w299, "PhoenixMotorControlDevRef"=w269) -> ()  [unwired: 7 in, 2 out]
  n147 = call <vilib>:"CTRE_Phoenix_MotorControl_RefNumRegistrySet.vi"("refnum name"=w308, "PhoenixMotorControlDevRef"=w275) -> ()  [unwired: 8 in, 2 out]
